vi "Write Waveforms.vi"(7 "Application Directory":path, 8 "Digital Format":string="Waveforms\\", 11 "Semiconductor Module Context":T1) -> (0 "error out":errorcluster)   [LabVIEW 2013]
uses:
  <vilib>/NI_TestStand_SemiconductorModule/NI_TestStand_Semiconductor_Module.lvlibp/PinMap/General/SemiconductorModuleContext.ctl
  <instrlib>/niHSDIO/niHSDIO.llb/niHSDIO Write Named Waveform From File (HWS).vi
  <vilib>/NI_TestStand_SemiconductorModule/NI_TestStand_Semiconductor_Module.lvlibp
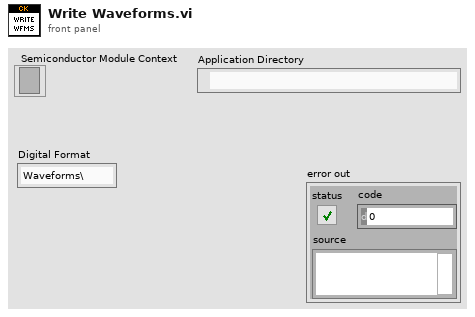
[diagram p1: front panel]
types:
  T1 = typedef "NI_TestStand_Semiconductor_Module.lvlibp/SemiconductorModuleContext.ctl" = refnum<k7>
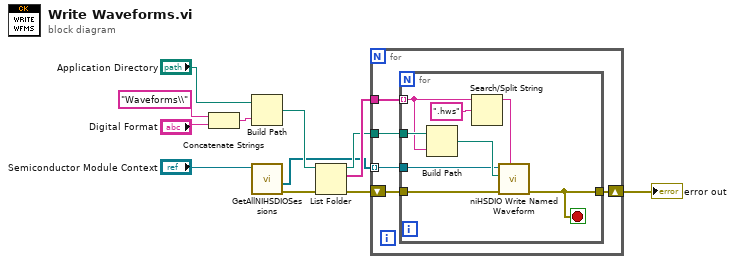
[diagram p0: block diagram]
diagram:
  n1 = Concatenate Strings("Waveforms\\" ("string"), "Digital Format") -> (w8:string)
  n2 = Build Path(base path="Application Directory", name or relative path=w8) -> (appended path=w5:path)
  n3 = call <vilib>:"GetAllNIHSDIOSessions.vi"("Semiconductor Module Context"="Semiconductor Module Context") -> ("error out"=w2:errorcluster, "Generation Sessions"=w4:refnum<k15>[])  [unwired: 7 in, 2 out]
  n4 = List Folder(path=w5, error in=w2) -> (path out=w6:path, filenames=w7:string[], error out=w1:errorcluster)  [unwired: 2 in, 1 out]
  n5 = for {
    tunnel: w7 -> [w17]
    tunnel: w6 -> [w16]
    tunnel: w4 -> [w15] mode=indexing
    shift-right: [w13] -> w3
    shift-left: w1 -> [w14]
    n6 = for {
      tunnel: w17 -> [w23] mode=indexing
      tunnel: w16 -> [w24]
      tunnel: w15 -> [w20]
      tunnel: w14 -> [w19]
      tunnel: [w18] -> w13
      stop <- w18 stop-if-true
      n7 = Build Path(base path=w24, name or relative path=w23) -> (appended path=w21:path)
      n8 = Search/Split String(string=w23, search string/char (-)=".hws") -> (substring before match=w22:string)  [unwired: 1 in, 2 out]
      n9 = call-poly <instrlib>:"niHSDIO Write Named Waveform.vi"("waveform name (default:\"\")"=w22, "error in (no error)"=w19, "file path"=w21, "instrument handle"=w20) -> ("error out"=w18:errorcluster)  [unwired: 5 in, 2 out]
    }
  }
  "error out" <- w3
